vi "Ignite Pilot.vi"(8 "error in (no error)":errorcluster, 10 "Indicator states in":T2 {"Time Count" format="%.2g"}, 11 "Runtime statuses in":T1) -> (0 "error out":errorcluster, 2 "Indicator states out":T2 {"Time Count" format="%.2g"}, 3 "Runtime statuses out":T1)   [LabVIEW 2014]
doc: "Checks runtime statuses. If Pre-Purge is complete logs Pilot ON event and starts alows Prove Pilot state"
uses:
  Controls/Boiler Status Indicators.ctl
  Controls/Boiler runtime status indicators.ctl
  Controls/Log file FGV action enum.ctl
  Controls/Log event enum.ctl
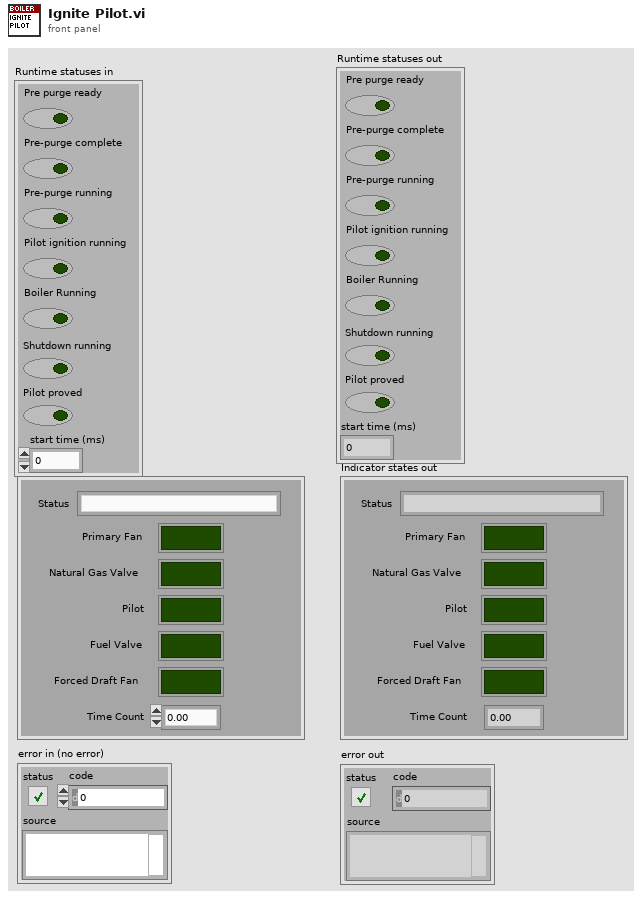
[diagram p1: front panel]
types:
  T1 = typedef "Boiler runtime status indicators.ctl" = cluster{"Pre purge ready":bool, "Pre-purge complete":bool, "Pre-purge running":bool, "Pilot ignition running":bool, "Boiler Running":bool, "Shutdown running":bool, "Pilot proved":bool, "start time (ms)":u32}
  T2 = typedef "Boiler Status Indicators.ctl" = cluster{"Status":string, "Primary Fan":bool, "Natural Gas Valve":bool, "Pilot":bool, "Fuel Valve":bool, "Forced Draft Fan":bool, "Time Count":dbl}
  T3 = typedef "Log event enum.ctl" = enum16{"Boiler Initialized", "Boiler Ready", "Start Pre-Purge", "Pre-Purge Complete", "Pilot ON", "Pilot proved", "Forced Draft Fan ON", "Boiler Running", "Start Shutdown Purge", "Shutdown Purge Complete"}
  T4 = typedef "Log file FGV action enum.ctl" = enum16{"open log file", "log event", "close log file"}
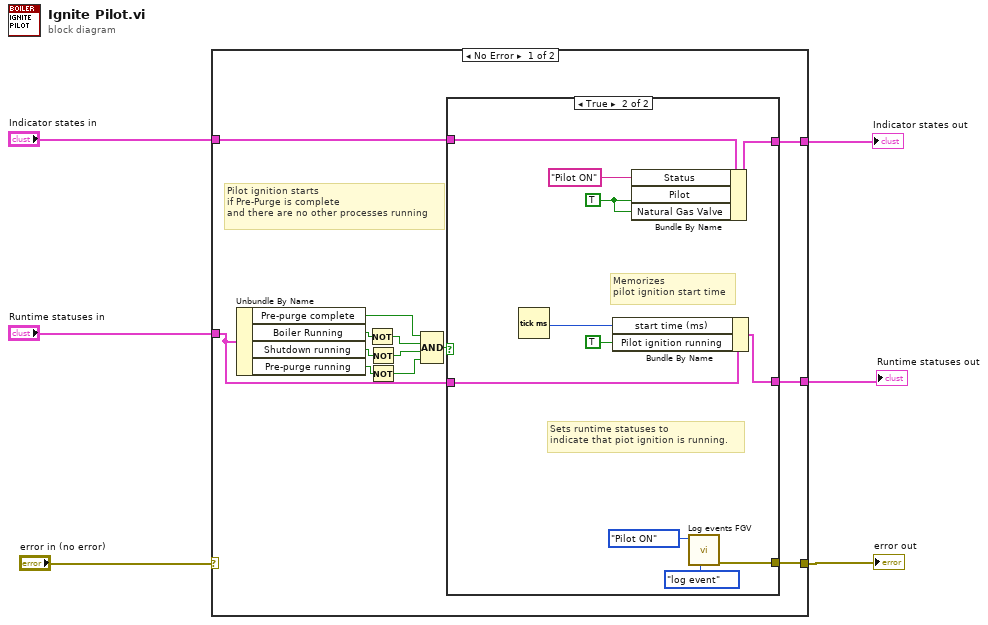
[diagram p0: block diagram]
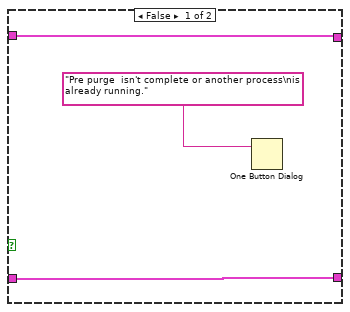
[diagram p2: hidden frame]
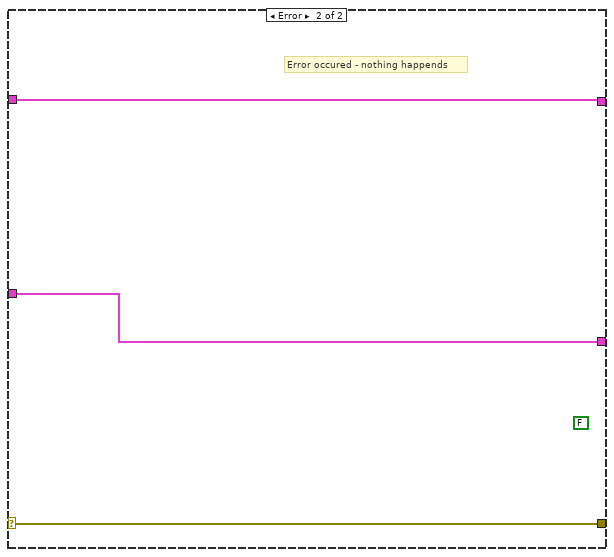
[diagram p3: hidden frame]
diagram:
  n1 = case shown="No Error" "error in (no error)" {
    selector: "error in (no error)" -> [_ w36]
    tunnel: [w7 w36] -> w5
    tunnel: "Runtime statuses in" -> [w13 w34]
    tunnel: "Indicator states in" -> [w15 w35]
    tunnel: [w14 w35] -> w2
    tunnel: [w12 w34] -> w1
    frame No Error {
      # "Pilot ignition starts\nif Pre-Purge is complete\nand there are no other processes running"
      n2 = Unbundle By Name(w13) -> ("Pre-purge complete"=w11:bool, "Boiler Running"=w18:bool, "Shutdown running"=w19:bool, "Pre-purge running"=w9:bool)
      n3 = Not(x=w18) -> (.not. x?=w10:bool)
      n4 = Not(x=w19) -> (.not. x?=w17:bool)
      n5 = Not(x=w9) -> (.not. x?=w8:bool)
      n6 = Compound Arithmetic op=AND(w11, w10, w17, w8) -> (w16:bool)
      n7 = case shown="True" w16 {
        tunnel: w15 -> [w22 w33]
        tunnel: [w22 w32] -> w14
        tunnel: w13 -> [w21 w30]
        tunnel: [w21 w29] -> w12
        tunnel: [_ w25] -> w7
        frame False {
          n8 = One Button Dialog(message="Pre purge  isn't complete or another process\nis already running.") -> ()  [unwired: 1 in, 1 out]
        }
        frame True {
          w27 = TRUE ("Primary Fan")
          # "Memorizes\npilot ignition start time"
          # "Sets runtime statuses to\nindicate that piot ignition is running."
          n9 = Tick Count (ms)() -> (millisecond timer value=w28:u32)
          n10 = Bundle By Name(cluster=w30, "start time (ms)"=w28, "Pilot ignition running"=TRUE) -> (w29:T1)
          n11 = Bundle By Name(cluster=w33, "Status"="Pilot ON", "Pilot"=w27, "Natural Gas Valve"=w27) -> (w32:T2)
          n12 = call "Log events FGV.vi"("action"=Log_file_FGV_action_enum."log event", "Log event"=Log_event_enum."Pilot ON") -> ("error out"=w25:errorcluster)  [unwired: 9 in]
        }
      }
    }
    frame Error {
      (unwired) FALSE
      # "Error occured - nothing happends"
    }
  }
  "Indicator states out" <- w2
  "error out" <- w5
  "Runtime statuses out" <- w1
